vi "getValFromVariant_double.vi"(8 "error in (no error)":errorcluster, 10 "name":string, 11 "variant":variant) -> (0 "error out":errorcluster, 3 "value":dbl)   [LabVIEW 2018]
doc: "Get the value from variant (double)."
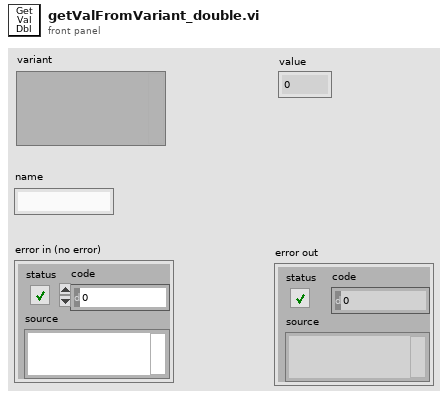
[diagram p1: front panel]
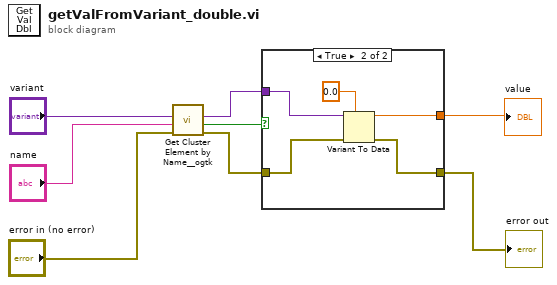
[diagram p0: block diagram]
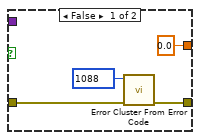
[diagram p2: hidden frame]
diagram:
  n1 = call <userlib>:"Get Cluster Element by Name__ogtk.vi"("error in (no error)"="error in (no error)", "Element Name"="name", "Cluster"="variant") -> ("error out"=w3:errorcluster, "found?"=w5:bool, "VElement"=w4:variant)  [unwired: 6 in]
  n2 = case shown="True" w5 {
    tunnel: w4 -> [_ w16]
    tunnel: w3 -> [w10 w15]
    tunnel: [w11 w14] -> w1
    tunnel: [0.0 w13] -> w2
    frame False {
      n3 = call <vilib>:"Error Cluster From Error Code.vi"("error in (no error)"=w10, "error code (0)"=1088) -> ("error out"=w11:errorcluster)  [unwired: 7 in]
    }
    frame True {
      n4 = Variant To Data(error in=w15, type=0.0, Variant=w16) -> (data=w13:dbl, error out=w14:errorcluster)
    }
  }
  "error out" <- w1
  "value" <- w2
